vi "test.vi"() -> ()   [LabVIEW 2018]
uses:
  <vilib>/Utility/file.llb/Read Delimited Spreadsheet (DBL).vi
panel:
  out "Array 2":u32[](array[numeric])
  out "Массив в формате boolean":bool[][](array[boolean])
  out "Массив регистров":string[][](array[string])
  out "array":i32[](array[numeric])
  out "Array":string[](array[string])
  out "Начальные данные":dbl[][](array[numeric])
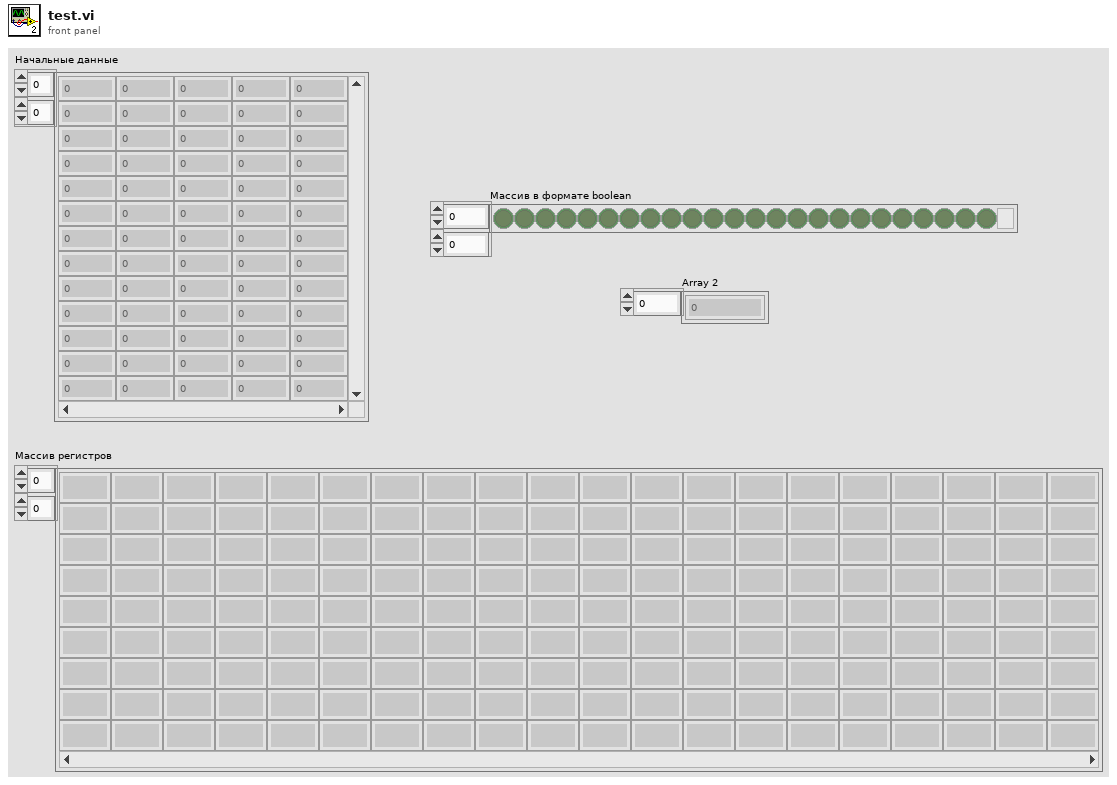
[diagram p1: front panel]
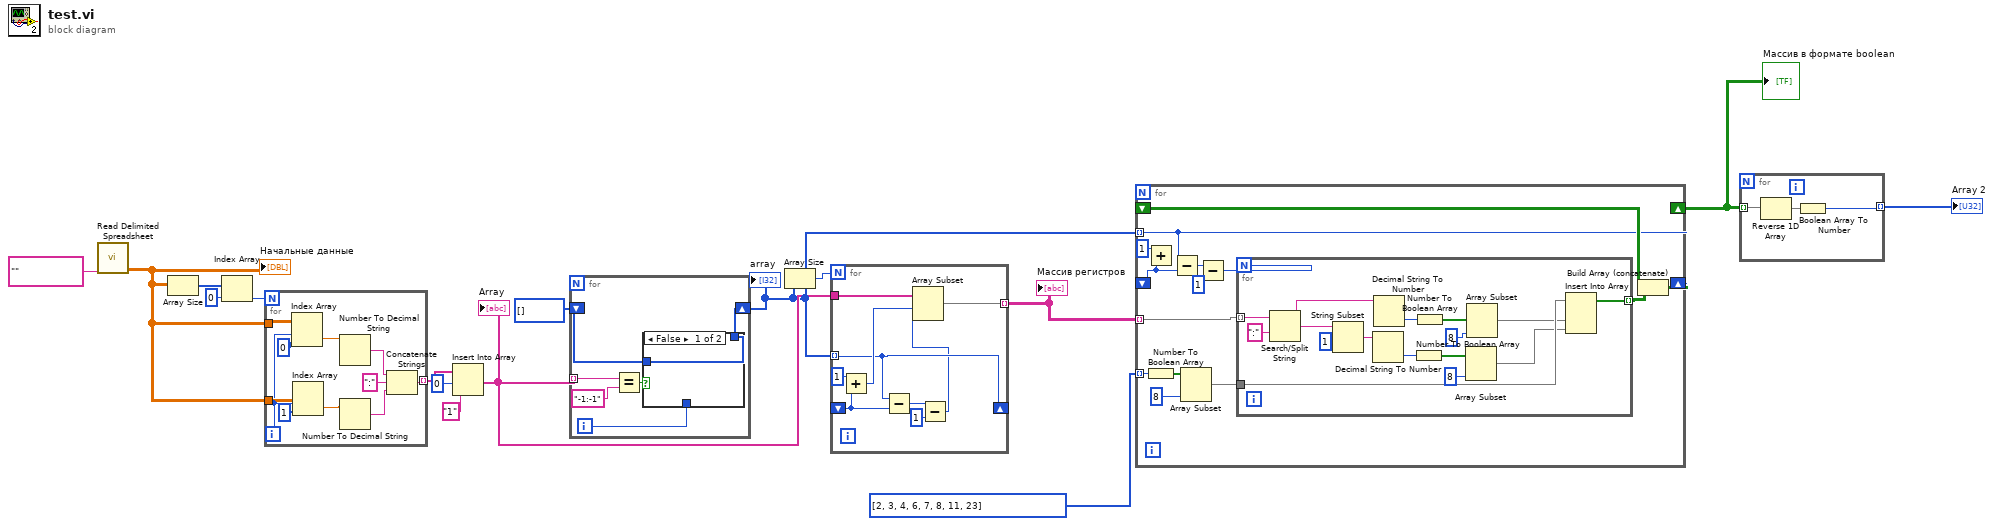
[diagram p0: block diagram]
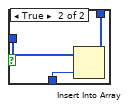
[diagram p2: hidden frame]
diagram:
  n1 = call-poly <vilib>:"Read Delimited Spreadsheet.vi"("delimiter (\\t)"="" ("delimiter (\\t)")) -> ("all rows"=w15:dbl[][])  [unwired: 9 in, 5 out]
  "Начальные данные" <- w15
  n2 = Array Size(array=w15) -> (size(s)=w14:i32[])
  n3 = Index Array(array=w14, index=0) -> (element=w12:i32)
  n4 = for {
    N: w12 -> [_]
    tunnel: w15 -> [w27]
    tunnel: w15 -> [w23]
    tunnel: [w21] -> w10 mode=indexing
    i -> [w22]
    n5 = Index Array(array=w23, index (row)=w22, index (col)=0 ("disabled index (col)")) -> (element=w18:dbl)
    n6 = Index Array(array=w27, index (row)=w22, index (col)=1 ("disabled index (col)")) -> (element=w17:dbl)
    n7 = Number To Decimal String(number=w18) -> (decimal integer string=w26:string)  [unwired: 1 in]
    n8 = Number To Decimal String(number=w17) -> (decimal integer string=w25:string)  [unwired: 1 in]
    n9 = Concatenate Strings(w26, ":" ("string"), w25) -> (w21:string)
  }
  n10 = Insert Into Array(array=w10, index=0, new element="1" ("new element/subarray")) -> (w7:string[])
  "Array" <- w7
  n11 = for {
    tunnel: w7 -> [w32] mode=indexing
    shift-right: [w28] -> w3
    shift-left: i32[] [] ("array") -> [w29]
    i -> [w30]
    n12 = Equal?(x=w32, y="-1:-1") -> (x = y?=w31:bool)
    n13 = case shown="False" w31 {
      tunnel: w30 -> [_ w37]
      tunnel: w29 -> [w34 w36]
      tunnel: [w34 w35] -> w28
      frame False {
      }
      frame True {
        n14 = Insert Into Array(array=w36, new element=w37) -> (w35:i32[])  [unwired: 1 in]
      }
    }
  }
  "array" <- w3
  n15 = Array Size(array=w3) -> (size(s)=w4:i32)
  n16 = for {
    N: w4 -> [_]
    tunnel: w3 -> [w41] mode=indexing
    tunnel: w7 -> [w46]
    shift-right: [w41] -> _
    shift-left: _ -> [w44]
    tunnel: [w45] -> w6 mode=indexing
    n17 = Add(x=1, y=w44) -> (x+y=w42:i32)
    n18 = Subtract(x=w41, y=w44) -> (x-y=w40:i32)
    n19 = Subtract(x=w40, y=1) -> (x-y=w39:i32)
    n20 = Array Subset(array=w46, index=w42, length=w39) -> (w45:string[])
  }
  "Массив регистров" <- w6
  n21 = for {
    tunnel: w6 -> [w55] mode=indexing
    tunnel: i32[] [2, 3, 4, 6, 7, 8, 11, 23] -> [w60] mode=indexing
    shift-right: [w53] -> w2
    shift-left: _ -> [w54]
    tunnel: w3 -> [w48] mode=indexing
    shift-right: [w48] -> _
    shift-left: _ -> [w47]
    n22 = Add(x=1, y=w47) -> ()  [unwired: 1 out]
    n23 = Number To Boolean Array(number=w60) -> (Boolean array=w57:bool[])
    n24 = Subtract(x=w48, y=w47) -> (x-y=w52:i32)
    n25 = Array Subset(array=w57, length=8) -> (w58:bool[])  [unwired: 1 in]
    n26 = Subtract(x=w52, y=1) -> (x-y=w50:i32)
    n27 = for {
      N: w50 -> [_]
      tunnel: w55 -> [w75] mode=indexing
      tunnel: w58 -> [w67]
      tunnel: [w68] -> w59 mode=indexing
      n28 = Search/Split String(string=w75, search string/char (-)=":") -> (substring before match=w69:string, match + rest of string=w74:string)  [unwired: 1 in, 1 out]
      n29 = String Subset(string=w74, offset (0)=1) -> (substring=w72:string)  [unwired: 1 in]
      n30 = Decimal String To Number(string=w72) -> (number=w71:i32)  [unwired: 2 in, 1 out]
      n31 = Decimal String To Number(string=w69) -> (number=w70:i32)  [unwired: 2 in, 1 out]
      n32 = Number To Boolean Array(number=w71) -> (Boolean array=w66:bool[])
      n33 = Number To Boolean Array(number=w70) -> (Boolean array=w65:bool[])
      n34 = Array Subset(array=w66, length=8) -> (w61:bool[])  [unwired: 1 in]
      n35 = Array Subset(array=w65, length=8) -> (w62:bool[])  [unwired: 1 in]
      n36 = Insert Into Array(array=w67, new element #1=w62, new element #2=w61) -> (w68:bool[])  [unwired: 1 in]
    }
    n37 = Build Array (concatenate)(w54, w59) -> (w53:bool[][])
  }
  "Массив в формате boolean" <- w2
  n38 = for {
    tunnel: w2 -> [w79] mode=indexing
    tunnel: [w77] -> w1 mode=indexing
    n39 = Reverse 1D Array(array=w79) -> (reversed array=w78:bool[])
    n40 = Boolean Array To Number(Boolean array=w78) -> (number=w77:u32)
  }
  "Array 2" <- w1
